vi "send_checkin_reply.vi"(5 "client id":string, 6 "cmd":T1=enum."CHECKOUT", 7 "start time":u32, 8 "error in (no error)":errorcluster, 9 "status":string, 10 "title":string, 11 "client tcp ref":refnum<k5>) -> (0 "error out":errorcluster, 2 "log string":string, 3 "client tcp ref out":refnum<k5>)   [LabVIEW 2020, in "librarian.lvclass"]
uses:
  librarian.lvclass
  shared/request--enum.ctl
  shared/message--cluster.ctl
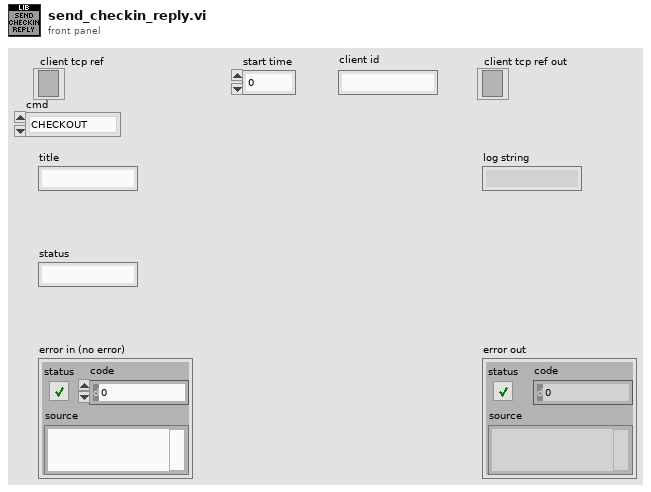
[diagram p1: front panel]
types:
  T1 = typedef "request--enum.ctl" = enum16{"CHECKIN", "CHECKOUT"}
  T2 = typedef "message--cluster.ctl" = cluster{"header":string, "cmd":T1, "title":string, "book":string}
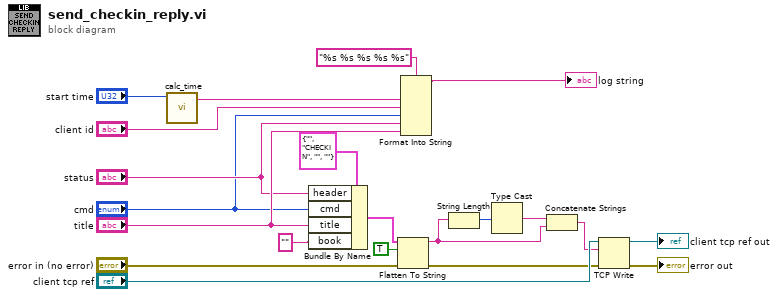
[diagram p0: block diagram]
diagram:
  n1 = call "calc_time.vi"("start time"="start time") -> ("String"=w11:string)  [unwired: 10 in]
  n2 = Bundle By Name(cluster=T2 {"header"="", "cmd"=enum."CHECKIN", "title"="", "book"=""} ("request"), "header"="status", "cmd"="cmd", "title"="title", "book"="") -> (w20:T2)
  n3 = Flatten To String(anything=w20, prepend array or string size? (T)=TRUE, error in (no error)="error in (no error)") -> (data string=w5:string, error out=w16:errorcluster)  [unwired: 1 in, 1 out]
  n4 = Format Into String(format string="%s %s %s %s %s", w11, "client id", "cmd", "status", "title") -> (resulting string=→"log string":string)  [unwired: 2 in, 1 out]
  n5 = String Length(string=w5) -> (length=w7:i32)
  n6 = Type Cast(x=w7) -> (*(type *) &x=w6:string)  [unwired: 1 in]
  n7 = Concatenate Strings(w6, w5) -> (w4:string)
  n8 = TCP Write(connection ID="client tcp ref", data in=w4, error in (no error)=w16) -> (connection ID out=→"client tcp ref out":refnum<k5>, error out=→"error out":errorcluster)  [unwired: 2 out]
